vi "Write Finish On.vi"(8 "error in (no error)":errorcluster, 10 "Finish On":T1, 11 "Repeater in":refnum<class "Repeater.lvclass">) -> (0 "error out":errorcluster, 3 "Repeater out":refnum<class "Repeater.lvclass">)   [LabVIEW 2021, in "BT.lvlib" / "Repeater.lvclass"]
uses:
  Repeater.lvclass
  Support/Finish On - Type.ctl
  Repeater.lvclass/Repeater.ctl
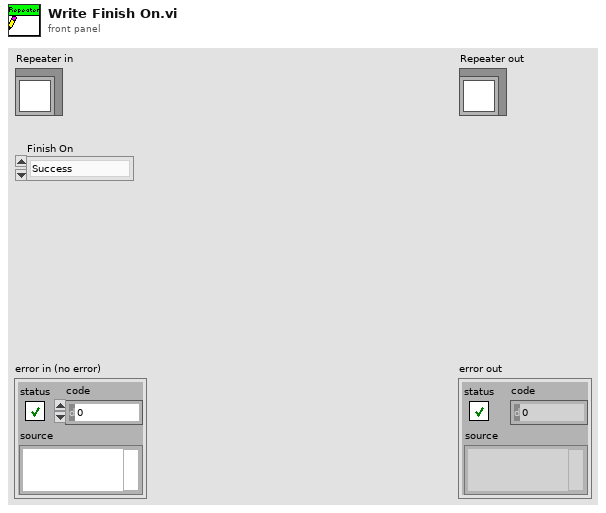
[diagram p1: front panel]
types:
  T1 = typedef "BT.lvlib/Repeater.lvclass/Finish On - Type.ctl" = enum16{"Success", "Failure", "Never"}
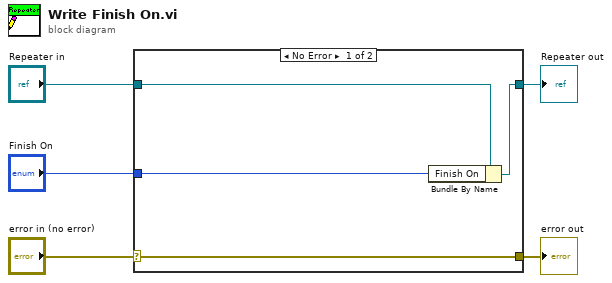
[diagram p0: block diagram]
diagram:
  n1 = case shown="No Error" "error in (no error)" {
    selector: "error in (no error)" -> [w9 w10]
    tunnel: [w9 w10] -> w4
    tunnel: [w7 w11] -> w2
    tunnel: "Repeater in" -> [w8 w11]
    tunnel: "Finish On" -> [w6 _]
    frame No Error {
      n2 = Bundle By Name(cluster=w8, "Finish On"=w6) -> (w7:refnum<class "Repeater.lvclass">)
    }
    frame Error {
    }
  }
  "error out" <- w4
  "Repeater out" <- w2
